vi "Multiplexer.vi"() -> ()   [LabVIEW 2021]
panel:
  out "O3":bool
  out "O2":bool
  out "O1":bool
  out "O0":bool
  out "output":bool
  in  "I3":bool
  in  "I2":bool
  in  "I1":bool
  in  "I0":bool
  in  "S1":bool
  in  "S0":bool
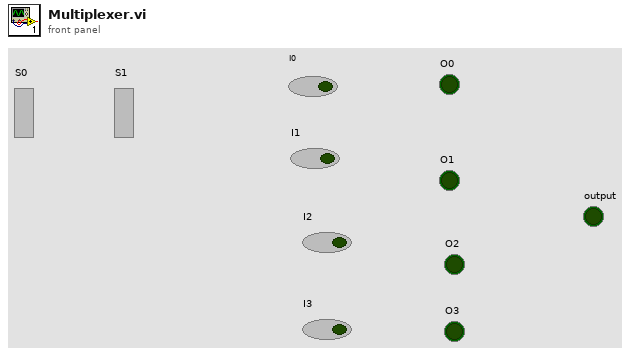
[diagram p1: front panel]
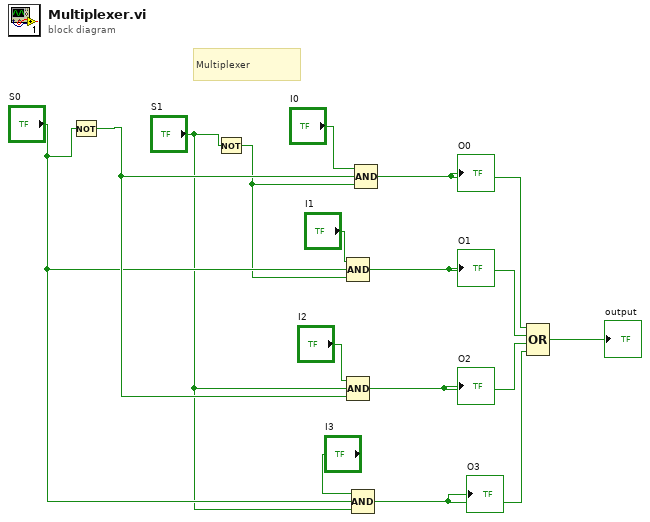
[diagram p0: block diagram]
diagram:
  # "Multiplexer"
  n1 = Not(x="S0") -> (.not. x?=w4:bool)
  n2 = Not(x="S1") -> (.not. x?=w2:bool)
  n3 = Compound Arithmetic op=AND("I1", "S0", w2) -> (w8:bool)
  "O1" <- w8
  n4 = Compound Arithmetic op=AND("I2", "S1", w4) -> (w7:bool)
  "O2" <- w7
  n5 = Compound Arithmetic op=AND("I3", "S0", "S1") -> (w6:bool)
  "O3" <- w6
  n6 = Compound Arithmetic op=AND("I0", w4, w2) -> (w5:bool)
  "O0" <- w5
  n7 = Compound Arithmetic op=OR(w5, w8, w7, w6) -> (→"output":bool)
